vi "Autotargeter.vi"(0 "Target":T3, 1 "Tip":T2, 3 "System of Reference Interface":T5, 4 "Refocus Step [um]":dbl=2.0, 5 "Max Distance [um]":dbl=20.0, 6 "Refocus threshold":dbl=0.2, 7 "Error In":errorcluster, 8 "Focus and Tracking":T4, 9 "Maximal Clearance [um]":dbl=15.0, 12 "Active":refnum<vi>, 13 "Minimal Clearance [um]":dbl=2.0, 14 "Dialog Indicator":refnum<vi>, 15 "Z direction":i8(ring)=-1 items=["Positive"=1, "Negative"=-1], 16 "Calibration":T6, 17 "Abort":refnum<vi>, 18 "Start Coordinates [pix]":refnum<vi>) -> (20 "Fail":bool, 21 "Scope Error":bool, 23 "Done":bool, 24 "Target Coordinates":T1, 27 "Error Out":errorcluster)   [LabVIEW 2012, in "Targeting Unit.lvlib"]
uses:
  Targeting Unit.lvlib
  <vilib>/Analysis/Matrix/Datatypes/RealMatrix.ctl
  <vilib>/Analysis/Matrix/NI_Matrix.lvlib
panel:
  in  "Contrast AVG frames number [unused]":i32=3
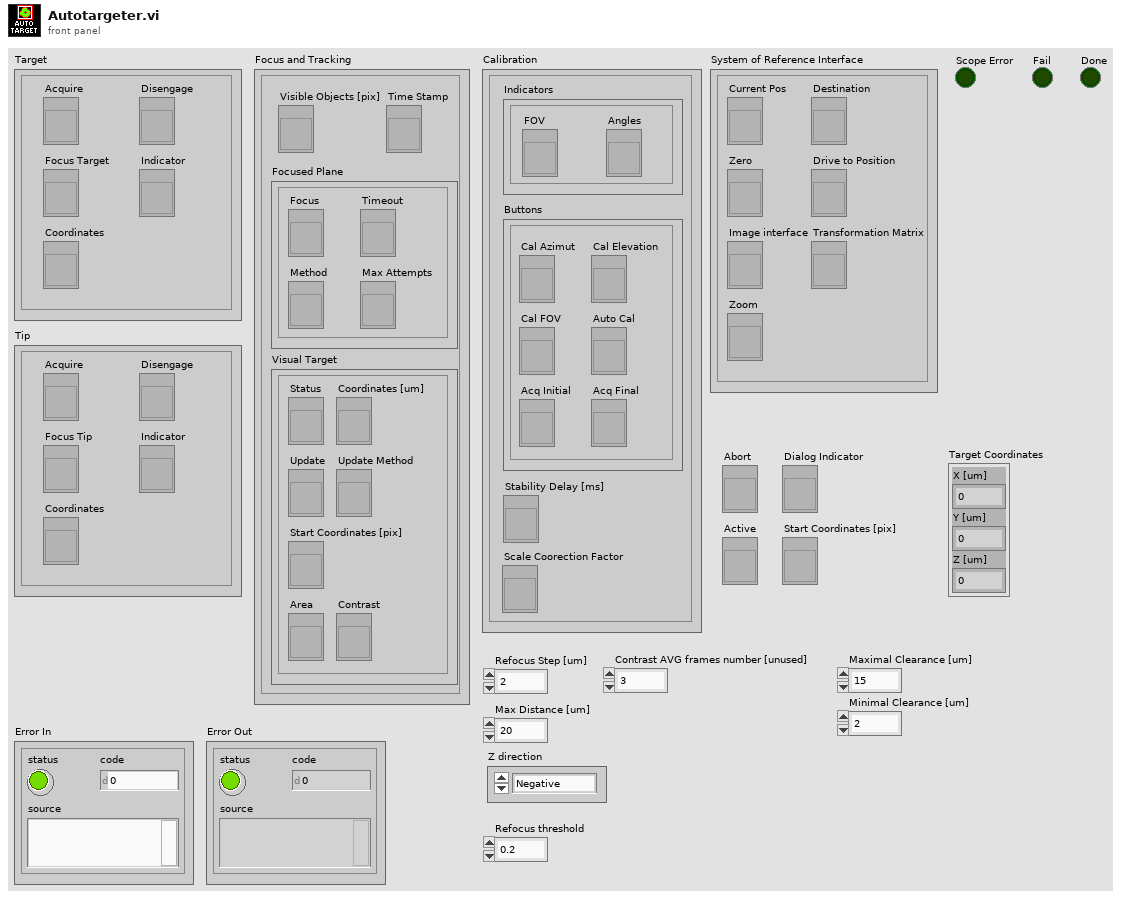
[diagram p1: front panel]
types:
  T1 = cluster{"X [um]":dbl, "Y [um]":dbl, "Z [um]":dbl}
  T2 = cluster{"Coordinates":refnum<vi>, "Acquire":refnum<vi>, "Disengage":refnum<vi>, "Indicator":refnum<vi>, "Focus Tip":refnum<vi>}
  T3 = cluster{"Coordinates":refnum<vi>, "Acquire":refnum<vi>, "Disengage":refnum<vi>, "Indicator":refnum<vi>, "Focus Target":refnum<vi>}
  T4 = cluster{"Focused Plane":cluster{"Focus":refnum<vi>, "Timeout":refnum<vi>, "Max Attempts":refnum<vi>, "Method":refnum<vi>}, "Time Stamp":refnum<vi>, "Visual Target":cluster{"Coordinates [um]":refnum<vi>, "Status":refnum<vi>, "Update":refnum<vi>, "Update Method":refnum<vi>, "Start Coordinates [pix]":refnum<vi>, "Area":refnum<vi>, "Contrast":refnum<vi>}, "Visible Objects [pix]":refnum<vi>}
  T5 = cluster{"Current Pos":refnum<vi>, "Image interface":refnum<vi>, "Transformation Matrix":refnum<vi>, "Zero":refnum<vi>, "Destination":refnum<vi>, "Drive to Position":refnum<vi>, "Zoom":refnum<vi>}
  T6 = cluster{"Indicators":cluster{"FOV":refnum<vi>, "Angles":refnum<vi>}, "Buttons":cluster{"Cal FOV":refnum<vi>, "Cal Azimut":refnum<vi>, "Cal Elevation":refnum<vi>, "Auto Cal":refnum<vi>, "Acq Initial":refnum<vi>, "Acq Final":refnum<vi>}, "Stability Delay [ms]":refnum<vi>, "Scale Coorection Factor":refnum<vi>}
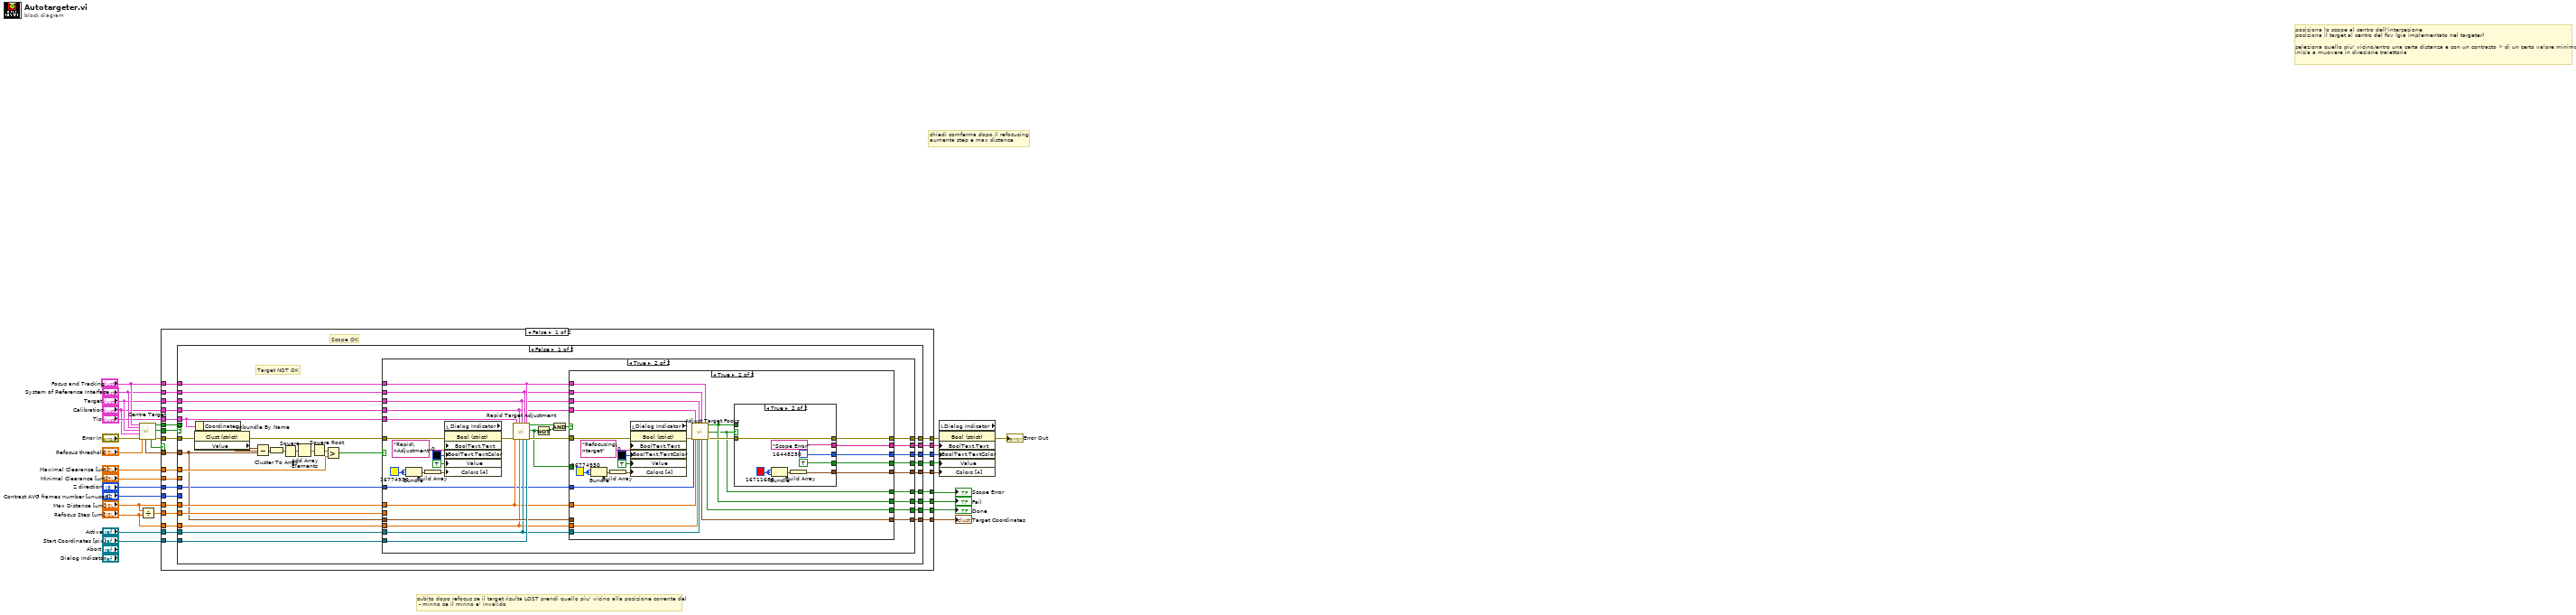
[diagram p0: block diagram]
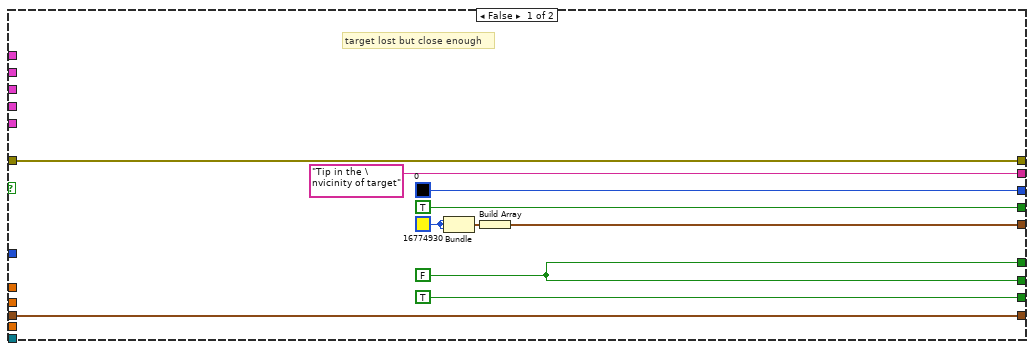
[diagram p2: hidden frame]
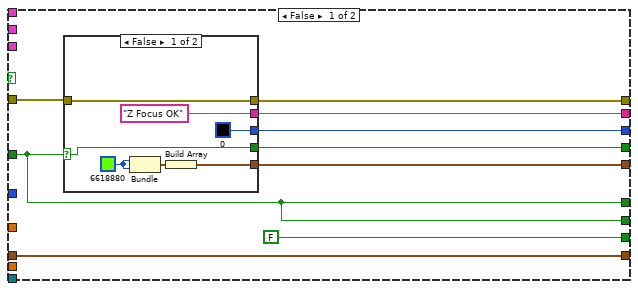
[diagram p3: hidden frame]
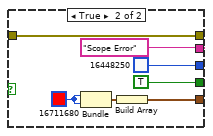
[diagram p4: hidden frame]
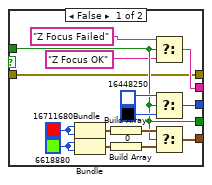
[diagram p5: hidden frame]
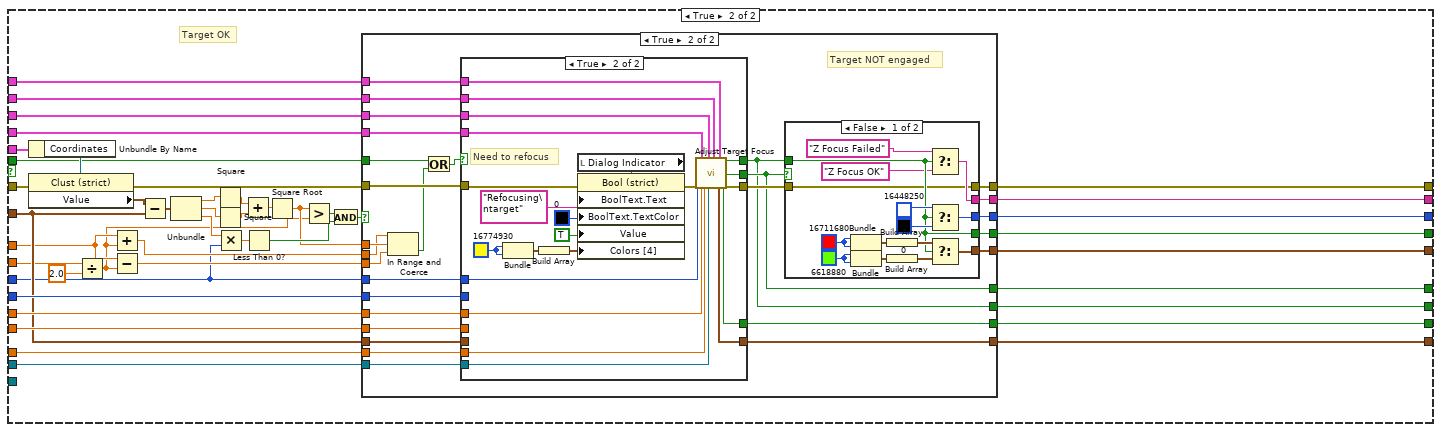
[diagram p6: hidden frame]
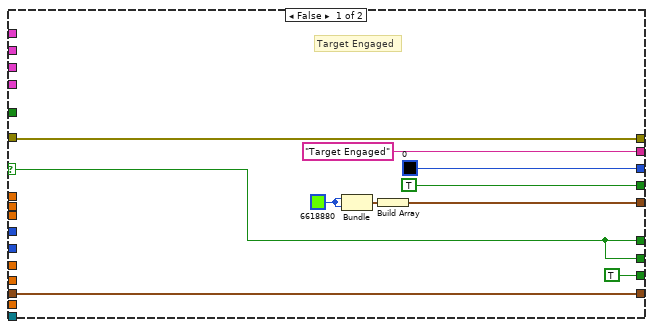
[diagram p7: hidden frame]
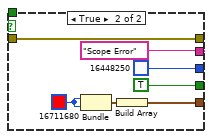
[diagram p8: hidden frame]
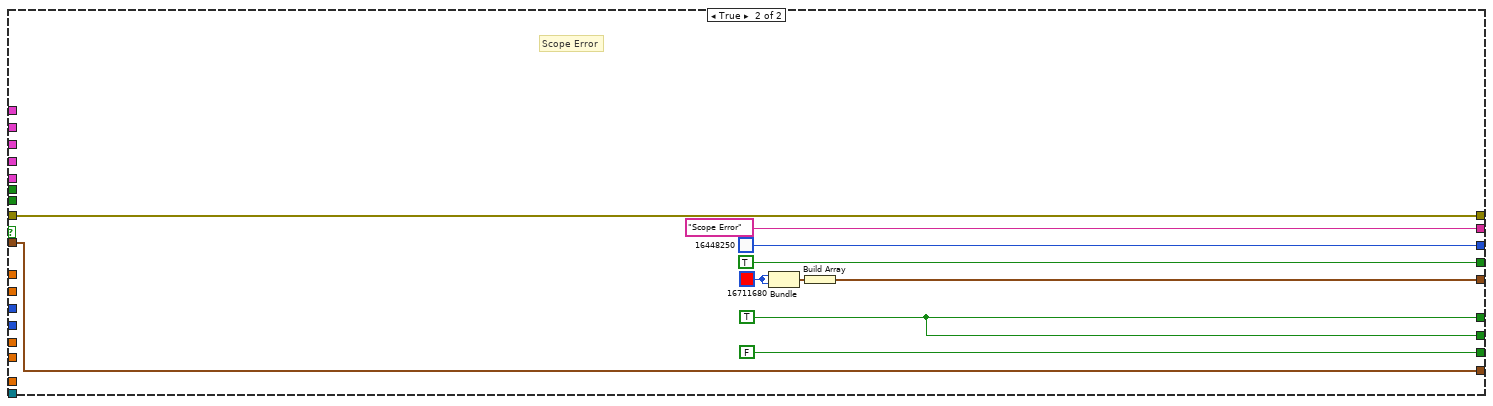
[diagram p10: hidden frame]
diagram:
  # "subito dopo refocus se il target risulta LOST prendi quello piu' vicino alla posizione corrente del \n - mirino se il mirino e' invalido"
  # "posiziona lo scope al centro dell'interzezione\nposiziona il target al centro del fov (gia implementato nel targeter)\n\nseleziona quello piu' vicino/entro una certa distanza e con un contrasto > di un certo valore minimo\ninizia a muovere in direzione traiettoria"
  # "chiedi comferma dopo il refocusing\naumenta step e max distance"
  n1 = call "Centre Target.vi"("Focus and Tracking"="Focus and Tracking", "Calibration"="Calibration", "System of Reference Interface"="System of Reference Interface", "Target"="Target", "error in (no error)"="Error In", "Refocus threshold"="Refocus threshold") -> ("Target Coordinates [um]"=w6:T1, "Need to refocus"=w15:bool, "Scope Error"=w3:bool, "Target OK"=w19:bool, "error out"=w18:errorcluster)  [unwired: 7 in, 2 out]
  n2 = Divide(x="Max Distance [um]", y="Refocus Step [um]") -> (x/y=w32:dbl)
  n3 = case shown="False" w3 {
    tunnel: w18 -> [w49 w340]
    tunnel: "Tip" -> [w59 _]
    tunnel: "System of Reference Interface" -> [w58 _]
    tunnel: "Target" -> [w57 _]
    tunnel: "Focus and Tracking" -> [w56 _]
    tunnel: w32 -> [w54 _]
    tunnel: [w45 w342] -> w31
    tunnel: [w44 w342] -> w30
    tunnel: "Contrast AVG frames number [unused]" -> [w55 _]
    tunnel: [w53 w341] -> w28
    tunnel: [w43 FALSE ("Error")] -> w27
    tunnel: "Maximal Clearance [um]" -> [w52 _]
    tunnel: "Minimal Clearance [um]" -> [w51 _]
    tunnel: "Max Distance [um]" -> [w50 _]
    tunnel: w19 -> [w35 _]
    tunnel: "Active" -> [w48 _]
    tunnel: "Refocus Step [um]" -> [w47 _]
    tunnel: w6 -> [w46 w341]
    tunnel: w15 -> [w42 _]
    tunnel: [w41 w340] -> w12
    tunnel: [w40 "Scope Error" ("Boolean Text.Text")] -> w11
    tunnel: [w39 u32 16448250] -> w10
    tunnel: [w38 TRUE ("Value")] -> w9
    tunnel: [w37 w336] -> w8
    tunnel: "Calibration" -> [w36 _]
    tunnel: "Z direction" -> [w34 _]
    tunnel: "Start Coordinates [pix]" -> [w33 _]
    frame False {
      # "Scope OK"
      n4 = case shown="False" w35 {
        tunnel: [w71 w221] -> w41
        tunnel: w49 -> [w64 w245]
        tunnel: w59 -> [w62 w244]
        tunnel: w58 -> [w90 w248]
        tunnel: w57 -> [w66 w223]
        tunnel: w56 -> [w75 w242]
        tunnel: w54 -> [w89 w250]
        tunnel: [w88 w247] -> w45
        tunnel: [w86 w241] -> w44
        tunnel: w55 -> [_ w249]
        tunnel: [w87 w246] -> w53
        tunnel: [w85 w240] -> w43
        tunnel: w52 -> [w79 w211]
        tunnel: w51 -> [_ w209]
        tunnel: w50 -> [w74 w228]
        tunnel: w48 -> [w72 w227]
        tunnel: w47 -> [w73 w215]
        tunnel: w46 -> [w65 w222]
        tunnel: w42 -> [_ w224]
        tunnel: [w70 w220] -> w40
        tunnel: [w69 w219] -> w39
        tunnel: [w68 w218] -> w38
        tunnel: [w67 w217] -> w37
        tunnel: w36 -> [w63 w216]
        tunnel: w34 -> [w60 w207]
        tunnel: w33 -> [w61 _]
        frame False {
          # "Target NOT OK"
          n5 = Unbundle By Name(w62) -> ("Coordinates"=w76:refnum<vi>)
          n6 = property class="Clust (strict)"(reference=w76, error in=w64) -> (error out=w77:errorcluster, "Value"=w84:T1)  [unwired: 1 out]
          n7 = Subtract(x=w84, y=w65) -> ()  [unwired: 1 out]
          n8 = Cluster To Array(cluster=w84) -> (array=w83:dbl[])
          n9 = Square(x=w83) -> (x^2=w82:dbl[])
          n10 = Add Array Elements(numeric array=w82) -> (sum=w81:dbl)
          n11 = Square Root(x=w81) -> (sqrt(x)=w80:dbl)
          n12 = Greater?(x=w80, y=w79) -> (0:w78:bool)
          n13 = case shown="True" w78 {
            tunnel: w90 -> [_ w113]
            tunnel: w89 -> [_ _]
            tunnel: w77 -> [w95 w126]
            tunnel: [w95 w120] -> w71
            tunnel: [w97 w119] -> w88
            tunnel: [w96 w123] -> w87
            tunnel: [w97 w110] -> w86
            tunnel: [TRUE w109] -> w85
            tunnel: w75 -> [_ w114]
            tunnel: w66 -> [_ w112]
            tunnel: w74 -> [_ w116]
            tunnel: w73 -> [_ w117]
            tunnel: w72 -> [_ w118]
            tunnel: w65 -> [w96 w122]
            tunnel: ["Tip in the \nvicinity of target" ("Boolean Text.Text") w108] -> w70
            tunnel: [u32 0 w107] -> w69
            tunnel: [TRUE ("Value") w106] -> w68
            tunnel: [w91 w105] -> w67
            tunnel: w63 -> [_ w111]
            tunnel: w62 -> [_ w125]
            tunnel: w61 -> [_ w124]
            tunnel: w60 -> [_ w115]
            frame False {
              w98 = u32 16774930
              w97 = FALSE ("Error")
              # "target lost but close enough"
              n14 = Bundle(w98, w98) -> (w99:cluster{u32, u32})  [unwired: 1 in]
              n15 = Build Array(w99) -> (w91:cluster{u32, u32}[])
            }
            frame True {
              w131 = u32 16774930
              n16 = Bundle(w131, w131) -> (w133:cluster{u32, u32})  [unwired: 1 in]
              n17 = Build Array(w133) -> (w128:cluster{u32, u32}[])
              n18 = local read "Dialog Indicator"() -> (w134:refnum<vi>)
              n19 = property class="Bool (strict)"(reference=w134, error in=w126, "BoolText.Text"="Rapid\nAdjustment" ("Boolean Text.Text"), "BoolText.TextColor"=u32 0, "Value"=TRUE, "Colors [4]"=w128) -> (error out=w127:errorcluster)  [unwired: 1 out]
              n20 = call "Rapid Target Adjustment.vi"("Focus and Tracking"=w114, "Calibration"=w111, "Target"=w112, "System of Reference Interface"=w113, "Tip"=w125, "Error In"=w127, "Step [um]"=w117, "Max Distance [um]"=w116, "Active"=w118, "Start Coordinates [pix]"=w124) -> ("Fail"=w103:bool, "Scope Error"=w101:bool, "Error Out"=w121:errorcluster)  [unwired: 5 in, 2 out]
              n21 = Not(x=w101) -> (.not. x?=w102:bool)
              n22 = And(x=w103, y=w102) -> (x .and. y?=w104:bool)
              n23 = case shown="True" w104 {
                tunnel: [w141 w164] -> w120
                tunnel: w116 -> [_ w176]
                tunnel: w115 -> [_ w175]
                tunnel: w118 -> [_ w174]
                tunnel: w113 -> [_ w173]
                tunnel: w114 -> [_ w172]
                tunnel: w121 -> [w140 w171]
                tunnel: w112 -> [_ w170]
                tunnel: [w143 w168] -> w123
                tunnel: w122 -> [w143 _]
                tunnel: [FALSE ("Aborted") w169] -> w109
                tunnel: w111 -> [_ w167]
                tunnel: w117 -> [_ w166]
                tunnel: [w139 w158] -> w119
                tunnel: [w139 w159] -> w110
                tunnel: w101 -> [w139 _]
                tunnel: [w138 w163] -> w108
                tunnel: [w137 w162] -> w107
                tunnel: [w136 w161] -> w106
                tunnel: [w135 w160] -> w105
                frame False {
                  n24 = case shown="False" w139 {
                    selector: w139 -> [w144 _]
                    tunnel: w140 -> [w148 w151]
                    tunnel: [w148 w151] -> w141
                    tunnel: [u32 0 u32 16448250] -> w137
                    tunnel: [w145 w152] -> w135
                    tunnel: [w144 TRUE ("Value")] -> w136
                    tunnel: ["Z Focus OK" ("Boolean Text.Text") "Scope Error" ("Boolean Text.Text")] -> w138
                    frame False {
                      w150 = u32 6618880
                      n25 = Bundle(w150, w150) -> (w149:cluster{u32, u32})  [unwired: 1 in]
                      n26 = Build Array(w149) -> (w145:cluster{u32, u32}[])
                    }
                    frame True {
                      w157 = u32 16711680
                      n27 = Bundle(w157, w157) -> (w156:cluster{u32, u32})  [unwired: 1 in]
                      n28 = Build Array(w156) -> (w152:cluster{u32, u32}[])
                    }
                  }
                }
                frame True {
                  w180 = u32 16774930
                  n29 = Bundle(w180, w180) -> (w182:cluster{u32, u32})  [unwired: 1 in]
                  n30 = Build Array(w182) -> (w177:cluster{u32, u32}[])
                  n31 = local read "Dialog Indicator"() -> (w183:refnum<vi>)
                  n32 = property class="Bool (strict)"(reference=w183, error in=w171, "BoolText.Text"="Refocusing\ntarget" ("Boolean Text.Text"), "BoolText.TextColor"=u32 0, "Value"=TRUE, "Colors [4]"=w177) -> (error out=w184:errorcluster)  [unwired: 1 out]
                  n33 = call "Adjust Target Focus.vi"("Target"=w170, "System of Reference Interface"=w173, "Focus and Tracking"=w172, "Calibration"=w167, "error in (no error)"=w184, "Distance [um]"=w176, "Refocus Step [um]"=w166, "Z direction"=w175, "Active"=w174) -> ("Focus Failed"=w159:bool, "Actual Coordinates [um]"=w168:T1, "Aborted"=w169:bool, "Scope Error"=w158:bool, "error out"=w165:errorcluster)  [unwired: 4 in, 2 out]
                  n34 = case shown="True" w158 {
                    tunnel: w165 -> [w185 w200]
                    tunnel: [w185 w200] -> w164
                    tunnel: w159 -> [w188 _]
                    tunnel: [w191 u32 16448250] -> w162
                    tunnel: [w190 w201] -> w160
                    tunnel: [w188 TRUE ("Value")] -> w161
                    tunnel: [w189 "Scope Error" ("Boolean Text.Text")] -> w163
                    frame False {
                      w194 = u32 6618880
                      w197 = u32 16711680
                      n35 = Bundle(w197, w197) -> (w196:cluster{u32, u32})  [unwired: 1 in]
                      n36 = Bundle(w194, w194) -> (w193:cluster{u32, u32})  [unwired: 1 in]
                      n37 = Build Array(w196) -> (w195:cluster{u32, u32}[])
                      n38 = Build Array(w193) -> (w192:cluster{u32, u32}[])
                      n39 = Select(t="Z Focus Failed" ("Boolean Text.Text"), s=w188, f="Z Focus OK" ("Boolean Text.Text")) -> (s? t:f=w189:string)
                      n40 = Select(t=u32 16448250, s=w188, f=u32 0) -> (s? t:f=w191:u32)
                      n41 = Select(t=w195, s=w188, f=w192) -> (s? t:f=w190:cluster{u32, u32}[])
                    }
                    frame True {
                      w206 = u32 16711680
                      n42 = Bundle(w206, w206) -> (w205:cluster{u32, u32})  [unwired: 1 in]
                      n43 = Build Array(w205) -> (w201:cluster{u32, u32}[])
                    }
                  }
                }
              }
            }
          }
        }
        frame True {
          # "Target OK"
          n44 = Unbundle By Name(w244) -> ("Coordinates"=w243:refnum<vi>)
          n45 = property class="Clust (strict)"(reference=w243, error in=w245) -> (error out=w226:errorcluster, "Value"=w225:T1)  [unwired: 1 out]
          n46 = Divide(x=w209, y=2.0) -> (x/y=w210:dbl)
          n47 = Add(x=w211, y=w210) -> (x+y=w212:dbl)
          n48 = Subtract(x=w211, y=w210) -> (x-y=w213:dbl)
          n49 = Subtract(x=w225, y=w222) -> (x-y=w239:T1)
          n50 = Unbundle(w239) -> ("X [um]"=w238:dbl, "Y [um]"=w237:dbl, "Z [um]"=w233:dbl)
          n51 = Square(x=w238) -> (x^2=w235:dbl)
          n52 = Square(x=w237) -> (x^2=w236:dbl)
          n53 = Multiply(x=w233, y=w207) -> (x*y=w230:dbl)
          n54 = Add(x=w235, y=w236) -> (x+y=w234:dbl)
          n55 = Less Than 0?(x=w230) -> (x < 0?=w229:bool)
          n56 = Square Root(x=w234) -> (sqrt(x)=w214:dbl)
          n57 = Greater?(x=w214, y=w210) -> (0:w232:bool)
          n58 = And(x=w232, y=w229) -> (x .and. y?=w231:bool)
          n59 = case shown="True" w231 {
            selector: w231 -> [w251 _]
            tunnel: w226 -> [w252 w279]
            tunnel: w242 -> [_ w282]
            tunnel: w250 -> [_ w288]
            tunnel: w249 -> [_ w287]
            tunnel: w248 -> [_ w281]
            tunnel: [w251 w280] -> w247
            tunnel: [w257 w276] -> w246
            tunnel: [w252 w271] -> w221
            tunnel: [w251 w270] -> w241
            tunnel: [TRUE w269] -> w240
            tunnel: w228 -> [_ w285]
            tunnel: w207 -> [_ w284]
            tunnel: w227 -> [_ w283]
            tunnel: w224 -> [_ w265]
            tunnel: w223 -> [_ w278]
            tunnel: w222 -> [w257 w277]
            tunnel: [w256 w275] -> w217
            tunnel: [TRUE ("Value") w274] -> w218
            tunnel: [u32 0 w273] -> w219
            tunnel: ["Target Engaged" ("Boolean Text.Text") w272] -> w220
            tunnel: w216 -> [_ w268]
            tunnel: w215 -> [_ w267]
            tunnel: w214 -> [_ w264]
            tunnel: w213 -> [_ w262]
            tunnel: w212 -> [_ w263]
            frame False {
              w260 = u32 6618880
              # "Target Engaged"
              n60 = Bundle(w260, w260) -> (w259:cluster{u32, u32})  [unwired: 1 in]
              n61 = Build Array(w259) -> (w256:cluster{u32, u32}[])
            }
            frame True {
              # "Target NOT engaged"
              n62 = In Range and Coerce(upper limit=w263, x=w264, lower limit=w262) -> (In Range?=w261:bool)  [unwired: 1 out]
              n63 = Or(x=w265, y=w261) -> (x .or. y?=w266:bool)
              n64 = case shown="True" w266 {
                selector: w266 -> [w311 _]
                tunnel: [w313 w327] -> w286
                tunnel: w288 -> [_ _]
                tunnel: [w311 w318] -> w280
                tunnel: [w311 w319] -> w270
                tunnel: w287 -> [_ _]
                tunnel: w285 -> [_ w326]
                tunnel: w284 -> [_ w325]
                tunnel: w283 -> [_ w324]
                tunnel: w281 -> [_ w323]
                tunnel: w282 -> [_ w322]
                tunnel: w279 -> [w313 w321]
                tunnel: w278 -> [_ w320]
                tunnel: [w312 w316] -> w276
                tunnel: w277 -> [w312 _]
                tunnel: [w311 w317] -> w269
                tunnel: w268 -> [_ w315]
                tunnel: w267 -> [_ w314]
                frame False {
                  # "Z focus ok"
                }
                frame True {
                  w331 = u32 16774930
                  # "Need to refocus"
                  n65 = Bundle(w331, w331) -> (w333:cluster{u32, u32})  [unwired: 1 in]
                  n66 = Build Array(w333) -> (w328:cluster{u32, u32}[])
                  n67 = local read "Dialog Indicator"() -> (w334:refnum<vi>)
                  n68 = property class="Bool (strict)"(reference=w334, error in=w321, "BoolText.Text"="Refocusing\ntarget" ("Boolean Text.Text"), "BoolText.TextColor"=u32 0, "Value"=TRUE, "Colors [4]"=w328) -> (error out=w335:errorcluster)  [unwired: 1 out]
                  n69 = call "Adjust Target Focus.vi"("Target"=w320, "System of Reference Interface"=w323, "Focus and Tracking"=w322, "Calibration"=w315, "error in (no error)"=w335, "Distance [um]"=w326, "Refocus Step [um]"=w314, "Z direction"=w325, "Active"=w324) -> ("Focus Failed"=w319:bool, "Actual Coordinates [um]"=w316:T1, "Aborted"=w317:bool, "Scope Error"=w318:bool, "error out"=w327:errorcluster)  [unwired: 4 in, 2 out]
                }
              }
              n70 = case shown="False" w280 {
                tunnel: w286 -> [w289 w304]
                tunnel: [w289 w304] -> w271
                tunnel: w270 -> [w292 _]
                tunnel: [w295 u32 16448250] -> w273
                tunnel: [w294 w305] -> w275
                tunnel: [w292 TRUE ("Value")] -> w274
                tunnel: [w293 "Scope Error" ("Boolean Text.Text")] -> w272
                frame False {
                  w298 = u32 6618880
                  w301 = u32 16711680
                  n71 = Bundle(w301, w301) -> (w300:cluster{u32, u32})  [unwired: 1 in]
                  n72 = Bundle(w298, w298) -> (w297:cluster{u32, u32})  [unwired: 1 in]
                  n73 = Build Array(w300) -> (w299:cluster{u32, u32}[])
                  n74 = Build Array(w297) -> (w296:cluster{u32, u32}[])
                  n75 = Select(t="Z Focus Failed" ("Boolean Text.Text"), s=w292, f="Z Focus OK" ("Boolean Text.Text")) -> (s? t:f=w293:string)
                  n76 = Select(t=u32 16448250, s=w292, f=u32 0) -> (s? t:f=w295:u32)
                  n77 = Select(t=w299, s=w292, f=w296) -> (s? t:f=w294:cluster{u32, u32}[])
                }
                frame True {
                  w310 = u32 16711680
                  n78 = Bundle(w310, w310) -> (w309:cluster{u32, u32})  [unwired: 1 in]
                  n79 = Build Array(w309) -> (w305:cluster{u32, u32}[])
                }
              }
            }
          }
        }
      }
    }
    frame True {
      w342 = TRUE ("Error")
      w344 = u32 16711680
      # "Scope Error"
      n80 = Bundle(w344, w344) -> (w345:cluster{u32, u32})  [unwired: 1 in]
      n81 = Build Array(w345) -> (w336:cluster{u32, u32}[])
    }
  }
  "Scope Error" <- w31
  "Fail" <- w30
  "Target Coordinates" <- w28
  "Done" <- w27
  n82 = local read "Dialog Indicator"() -> (w13:refnum<vi>)
  n83 = property class="Bool (strict)"(reference=w13, error in=w12, "BoolText.Text"=w11, "BoolText.TextColor"=w10, "Value"=w9, "Colors [4]"=w8) -> (error out=→"Error Out":errorcluster)  [unwired: 1 out]
